vi "Magazine_Hardware_Begin.vi"(8 "error in":errorcluster) -> (0 "error out":errorcluster)   [LabVIEW 2020]
uses:
  <vilib>/Rock Robotics/SystemInterfaces/AI/FPGA_AIChannel.ctl
  <vilib>/Rock Robotics/WPI/ThirdParty/Phoenix-LabVIEW/Motor Controller/Controls/CTRE_Phoenix_MotorControl_NeutralMode.ctl
  <vilib>/Rock Robotics/WPI/ThirdParty/Phoenix-LabVIEW/Motor Controller/Controls/CTRE_Phoenix_MotorControl_StatusFrameEnhanced.ctl
  Globals/Magazine_Globals.vi
panel:
  out "appended array":u32[](array[numeric])
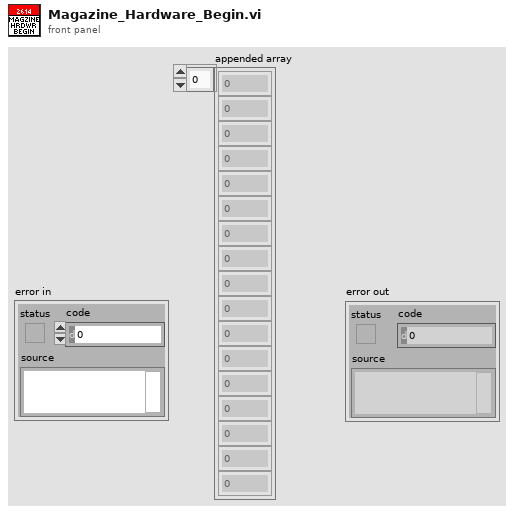
[diagram p1: front panel]
types:
  T1 = typedef "CTRE_Phoenix_MotorControl_StatusFrameEnhanced.ctl" = u16
  T2 = typedef "CTRE_Phoenix_MotorControl_NeutralMode.ctl" = enum8{"EEPROMSetting", "Override to Coast", "Override to Brake"}
  T3 = typedef "FPGA_AIChannel.ctl" = enum8{"AI 0", "AI 1", "AI 2", "AI 3", "AI MXP 0", "AI MXP 1", "AI MXP 2", "AI MXP 3", "Invalid"}
  T4 = typedef "WPI_MotorControlDeviceRef.ctl" = cluster{"DeviceStatus":errorcluster, "Type":T5, "PWM":cluster{"PWM Channel":T6, "DeadBand":T7}, "CAN":cluster{"Device Number":u8, "SetOutput VI Ref":variant, "GetOutput VI Ref":variant, "Enable VI Ref":variant, "Disable VI Ref":variant, "Data":variant}, "Invert":bool, "DIO PWM":cluster{"PWM \"Enable\" Channel":T6, "DIOChannel":T8, "PWM Rate":dbl}}
  T5 = typedef "WPI_MotorControlType.ctl" = enum16{"PWM", "CAN", "DIO PWM"}
  T6 = typedef "FPGA_DIOPWMChannel.ctl" = enum8{"PWM 0", "PWM 1", "PWM 2", "PWM 3", "PWM 4", "PWM 5", "PWM 6", "PWM 7", "PWM 8", "PWM 9", "PWM MXP 0", "PWM MXP 1", "PWM MXP 2", "PWM MXP 3", "PWM MXP 4", "PWM MXP 5", "PWM MXP 6", "PWM MXP 7", "PWM MXP 8", "PWM MXP 9", "Invalid"}
  T7 = typedef "WPI_PWMDeadband.ctl" = cluster{"Name":string, "maxPositivePwm":i32, "minPositivePwm":i32, "centerPwm":i32, "maxNegativePwm":i32, "minNegativePwm":i32, "angularRange":u16}
  T8 = typedef "FPGA_DIOChannel.ctl" = enum8{"DIO 0", "DIO 1", "DIO 2", "DIO 3", "DIO 4", "DIO 5", "DIO 6", "DIO 7", "DIO 8", "DIO 9", "DIO MXP 0", "DIO MXP 1", "DIO MXP 2", "DIO MXP 3", "DIO MXP 4", "DIO MXP 5", "DIO MXP 6", "DIO MXP 7", "DIO MXP 8", "DIO MXP 9", "DIO MXP 10", "DIO MXP 11", "DIO MXP 12", "DIO MXP 13", "DIO MXP 14", "DIO MXP 15", "SPI Port CS1", "SPI Port CS2", "SPI Port CS3", "SPI Port MISO", "SPI Port MOSI", "Invalid"}
  T9 = typedef "WPI_AnalogChannelDevRef.ctl" = cluster{"DevStatus":errorcluster, "Analog Channel":T3}
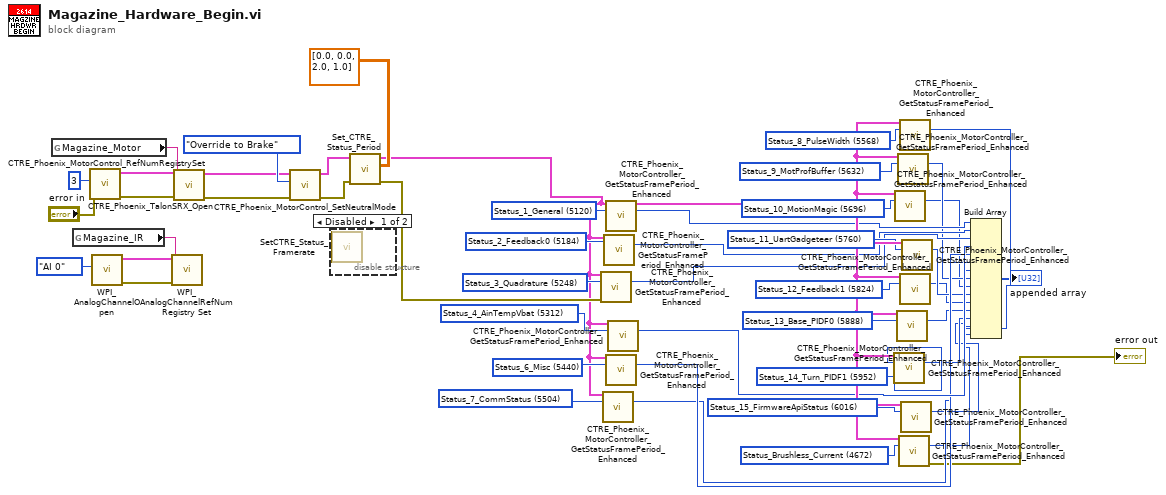
[diagram p0: block diagram]
diagram:
  w26 = T1 4672 items=["Status_1_General"=5120, "Status_2_Feedback0"=5184, "Status_3_Quadrature"=5248, "Status_4_AinTempVbat"=5312, "Status_6_Misc"=5440, "Status_7_CommStatus"=5504, "Status_8_PulseWidth"=5568, "Status_9_MotProfBuffer"=5632, "Status_10_MotionMagic"=5696, "Status_11_UartGadgeteer"=5760, "Status_12_Feedback1"=5824, "Status_13_Base_PIDF0"=5888, "Status_14_Turn_PIDF1"=5952, "Status_15_FirmwareApiStatus"=6016, "Status_Brushless_Current"=4672] ("Status Frame")
  w27 = T1 6016 items=["Status_1_General"=5120, "Status_2_Feedback0"=5184, "Status_3_Quadrature"=5248, "Status_4_AinTempVbat"=5312, "Status_6_Misc"=5440, "Status_7_CommStatus"=5504, "Status_8_PulseWidth"=5568, "Status_9_MotProfBuffer"=5632, "Status_10_MotionMagic"=5696, "Status_11_UartGadgeteer"=5760, "Status_12_Feedback1"=5824, "Status_13_Base_PIDF0"=5888, "Status_14_Turn_PIDF1"=5952, "Status_15_FirmwareApiStatus"=6016, "Status_Brushless_Current"=4672] ("Status Frame")
  w28 = T1 5952 items=["Status_1_General"=5120, "Status_2_Feedback0"=5184, "Status_3_Quadrature"=5248, "Status_4_AinTempVbat"=5312, "Status_6_Misc"=5440, "Status_7_CommStatus"=5504, "Status_8_PulseWidth"=5568, "Status_9_MotProfBuffer"=5632, "Status_10_MotionMagic"=5696, "Status_11_UartGadgeteer"=5760, "Status_12_Feedback1"=5824, "Status_13_Base_PIDF0"=5888, "Status_14_Turn_PIDF1"=5952, "Status_15_FirmwareApiStatus"=6016, "Status_Brushless_Current"=4672] ("Status Frame")
  w29 = T1 5888 items=["Status_1_General"=5120, "Status_2_Feedback0"=5184, "Status_3_Quadrature"=5248, "Status_4_AinTempVbat"=5312, "Status_6_Misc"=5440, "Status_7_CommStatus"=5504, "Status_8_PulseWidth"=5568, "Status_9_MotProfBuffer"=5632, "Status_10_MotionMagic"=5696, "Status_11_UartGadgeteer"=5760, "Status_12_Feedback1"=5824, "Status_13_Base_PIDF0"=5888, "Status_14_Turn_PIDF1"=5952, "Status_15_FirmwareApiStatus"=6016, "Status_Brushless_Current"=4672] ("Status Frame")
  w34 = T1 5824 items=["Status_1_General"=5120, "Status_2_Feedback0"=5184, "Status_3_Quadrature"=5248, "Status_4_AinTempVbat"=5312, "Status_6_Misc"=5440, "Status_7_CommStatus"=5504, "Status_8_PulseWidth"=5568, "Status_9_MotProfBuffer"=5632, "Status_10_MotionMagic"=5696, "Status_11_UartGadgeteer"=5760, "Status_12_Feedback1"=5824, "Status_13_Base_PIDF0"=5888, "Status_14_Turn_PIDF1"=5952, "Status_15_FirmwareApiStatus"=6016, "Status_Brushless_Current"=4672] ("Status Frame")
  w30 = T1 5760 items=["Status_1_General"=5120, "Status_2_Feedback0"=5184, "Status_3_Quadrature"=5248, "Status_4_AinTempVbat"=5312, "Status_6_Misc"=5440, "Status_7_CommStatus"=5504, "Status_8_PulseWidth"=5568, "Status_9_MotProfBuffer"=5632, "Status_10_MotionMagic"=5696, "Status_11_UartGadgeteer"=5760, "Status_12_Feedback1"=5824, "Status_13_Base_PIDF0"=5888, "Status_14_Turn_PIDF1"=5952, "Status_15_FirmwareApiStatus"=6016, "Status_Brushless_Current"=4672] ("Status Frame")
  w35 = T1 5696 items=["Status_1_General"=5120, "Status_2_Feedback0"=5184, "Status_3_Quadrature"=5248, "Status_4_AinTempVbat"=5312, "Status_6_Misc"=5440, "Status_7_CommStatus"=5504, "Status_8_PulseWidth"=5568, "Status_9_MotProfBuffer"=5632, "Status_10_MotionMagic"=5696, "Status_11_UartGadgeteer"=5760, "Status_12_Feedback1"=5824, "Status_13_Base_PIDF0"=5888, "Status_14_Turn_PIDF1"=5952, "Status_15_FirmwareApiStatus"=6016, "Status_Brushless_Current"=4672] ("Status Frame")
  w31 = T1 5632 items=["Status_1_General"=5120, "Status_2_Feedback0"=5184, "Status_3_Quadrature"=5248, "Status_4_AinTempVbat"=5312, "Status_6_Misc"=5440, "Status_7_CommStatus"=5504, "Status_8_PulseWidth"=5568, "Status_9_MotProfBuffer"=5632, "Status_10_MotionMagic"=5696, "Status_11_UartGadgeteer"=5760, "Status_12_Feedback1"=5824, "Status_13_Base_PIDF0"=5888, "Status_14_Turn_PIDF1"=5952, "Status_15_FirmwareApiStatus"=6016, "Status_Brushless_Current"=4672] ("Status Frame")
  w36 = T1 5568 items=["Status_1_General"=5120, "Status_2_Feedback0"=5184, "Status_3_Quadrature"=5248, "Status_4_AinTempVbat"=5312, "Status_6_Misc"=5440, "Status_7_CommStatus"=5504, "Status_8_PulseWidth"=5568, "Status_9_MotProfBuffer"=5632, "Status_10_MotionMagic"=5696, "Status_11_UartGadgeteer"=5760, "Status_12_Feedback1"=5824, "Status_13_Base_PIDF0"=5888, "Status_14_Turn_PIDF1"=5952, "Status_15_FirmwareApiStatus"=6016, "Status_Brushless_Current"=4672] ("Status Frame")
  w6 = T1 5504 items=["Status_1_General"=5120, "Status_2_Feedback0"=5184, "Status_3_Quadrature"=5248, "Status_4_AinTempVbat"=5312, "Status_6_Misc"=5440, "Status_7_CommStatus"=5504, "Status_8_PulseWidth"=5568, "Status_9_MotProfBuffer"=5632, "Status_10_MotionMagic"=5696, "Status_11_UartGadgeteer"=5760, "Status_12_Feedback1"=5824, "Status_13_Base_PIDF0"=5888, "Status_14_Turn_PIDF1"=5952, "Status_15_FirmwareApiStatus"=6016, "Status_Brushless_Current"=4672] ("Status Frame")
  w32 = T1 5440 items=["Status_1_General"=5120, "Status_2_Feedback0"=5184, "Status_3_Quadrature"=5248, "Status_4_AinTempVbat"=5312, "Status_6_Misc"=5440, "Status_7_CommStatus"=5504, "Status_8_PulseWidth"=5568, "Status_9_MotProfBuffer"=5632, "Status_10_MotionMagic"=5696, "Status_11_UartGadgeteer"=5760, "Status_12_Feedback1"=5824, "Status_13_Base_PIDF0"=5888, "Status_14_Turn_PIDF1"=5952, "Status_15_FirmwareApiStatus"=6016, "Status_Brushless_Current"=4672] ("Status Frame")
  w33 = T1 5312 items=["Status_1_General"=5120, "Status_2_Feedback0"=5184, "Status_3_Quadrature"=5248, "Status_4_AinTempVbat"=5312, "Status_6_Misc"=5440, "Status_7_CommStatus"=5504, "Status_8_PulseWidth"=5568, "Status_9_MotProfBuffer"=5632, "Status_10_MotionMagic"=5696, "Status_11_UartGadgeteer"=5760, "Status_12_Feedback1"=5824, "Status_13_Base_PIDF0"=5888, "Status_14_Turn_PIDF1"=5952, "Status_15_FirmwareApiStatus"=6016, "Status_Brushless_Current"=4672] ("Status Frame")
  w7 = T1 5248 items=["Status_1_General"=5120, "Status_2_Feedback0"=5184, "Status_3_Quadrature"=5248, "Status_4_AinTempVbat"=5312, "Status_6_Misc"=5440, "Status_7_CommStatus"=5504, "Status_8_PulseWidth"=5568, "Status_9_MotProfBuffer"=5632, "Status_10_MotionMagic"=5696, "Status_11_UartGadgeteer"=5760, "Status_12_Feedback1"=5824, "Status_13_Base_PIDF0"=5888, "Status_14_Turn_PIDF1"=5952, "Status_15_FirmwareApiStatus"=6016, "Status_Brushless_Current"=4672] ("Status Frame")
  w8 = T1 5184 items=["Status_1_General"=5120, "Status_2_Feedback0"=5184, "Status_3_Quadrature"=5248, "Status_4_AinTempVbat"=5312, "Status_6_Misc"=5440, "Status_7_CommStatus"=5504, "Status_8_PulseWidth"=5568, "Status_9_MotProfBuffer"=5632, "Status_10_MotionMagic"=5696, "Status_11_UartGadgeteer"=5760, "Status_12_Feedback1"=5824, "Status_13_Base_PIDF0"=5888, "Status_14_Turn_PIDF1"=5952, "Status_15_FirmwareApiStatus"=6016, "Status_Brushless_Current"=4672] ("Status Frame")
  w37 = T1 5120 items=["Status_1_General"=5120, "Status_2_Feedback0"=5184, "Status_3_Quadrature"=5248, "Status_4_AinTempVbat"=5312, "Status_6_Misc"=5440, "Status_7_CommStatus"=5504, "Status_8_PulseWidth"=5568, "Status_9_MotProfBuffer"=5632, "Status_10_MotionMagic"=5696, "Status_11_UartGadgeteer"=5760, "Status_12_Feedback1"=5824, "Status_13_Base_PIDF0"=5888, "Status_14_Turn_PIDF1"=5952, "Status_15_FirmwareApiStatus"=6016, "Status_Brushless_Current"=4672] ("Status Frame")
  n1 = global read "Magazine_Globals.vi" "Magazine_Motor"() -> (w50:string)
  n2 = global read "Magazine_Globals.vi" "Magazine_IR"() -> (w44:string)
  n3 = call <vilib>:"CTRE_Phoenix_TalonSRX_Open.vi"("error in"="error in", "Device Number"=u8 3) -> ("error out"=w48:errorcluster, "PhoenixMotorControlDevRef"=w49:T4)  [unwired: 8 in]
  n4 = call <vilib>:"WPI_AnalogChannelOpen.vi"("Analog Channel"=FPGA_AIChannel."AI 0") -> ("error out"=w45:errorcluster, "AIDeviceRef"=w46:T9)  [unwired: 9 in]
  n5 = call <vilib>:"WPI_AnalogChannelRefNum Registry Set.vi"("error in (no error)"=w45, "refnum name"=w44, "AIDeviceRef"=w46) -> ()  [unwired: 7 in, 2 out]
  n6 = call <vilib>:"CTRE_Phoenix_MotorControl_RefNumRegistrySet.vi"("error in (no error)"=w48, "refnum name"=w50, "PhoenixMotorControlDevRef"=w49) -> ("error out"=w39:errorcluster, "PhoenixMotorControlDevRef"=w40:T4)  [unwired: 7 in]
  n7 = call <vilib>:"CTRE_Phoenix_MotorControl_SetNeutralMode.vi"("error in (no error)"=w39, "Motor Control Neutral Mode"=CTRE_Phoenix_MotorControl_NeutralMode."Override to Brake", "PhoenixMotorControlDevRef"=w40) -> ("error out"=w3:errorcluster, "PhoenixMotorControlDevRef"=w4:T4)  [unwired: 7 in]
  n8 = disable-structure shown="Disabled" {
    frame Disabled {
      n9 = call "SetCTRE_Status_Framerate.vi"() -> ()  [unwired: 10 in, 2 out]
    }
    frame Enabled {
    }
  }
  n10 = call "Set_CTRE_Status_Period.vi"("error in (no error)"=w3, "Frame Settings"=dbl[][] [[0.0], [0.0], [2.0], [1.0]], "PhoenixMotorControlDevRef"=w4) -> ("error out"=w2:errorcluster, "PhoenixMotorControlDevRef 2"=w1:T4)  [unwired: 7 in]
  n11 = call <vilib>:"CTRE_Phoenix_MotorController_GetStatusFramePeriod_Enhanced.vi"("PhoenixMotorControlDevRef"=w1, "Status Frame"=w7, "error in"=w2) -> ("periodMs"=w23:u32)  [unwired: 10 in, 2 out]
  n12 = call <vilib>:"CTRE_Phoenix_MotorController_GetStatusFramePeriod_Enhanced.vi"("PhoenixMotorControlDevRef"=w1, "Status Frame"=w6) -> ("periodMs"=w20:u32)  [unwired: 11 in, 2 out]
  n13 = call <vilib>:"CTRE_Phoenix_MotorController_GetStatusFramePeriod_Enhanced.vi"("PhoenixMotorControlDevRef"=w1, "Status Frame"=w8) -> ("periodMs"=w24:u32)  [unwired: 11 in, 2 out]
  n14 = call <vilib>:"CTRE_Phoenix_MotorController_GetStatusFramePeriod_Enhanced.vi"("PhoenixMotorControlDevRef"=w1, "Status Frame"=w37) -> ("PhoenixMotorControlDevRef"=w38:T4, "periodMs"=w25:u32)  [unwired: 11 in, 1 out]
  n15 = call <vilib>:"CTRE_Phoenix_MotorController_GetStatusFramePeriod_Enhanced.vi"("PhoenixMotorControlDevRef"=w1, "Status Frame"=w32) -> ("periodMs"=w21:u32)  [unwired: 11 in, 2 out]
  n16 = call <vilib>:"CTRE_Phoenix_MotorController_GetStatusFramePeriod_Enhanced.vi"("PhoenixMotorControlDevRef"=w1, "Status Frame"=w33) -> ("periodMs"=w22:u32)  [unwired: 11 in, 2 out]
  n17 = call <vilib>:"CTRE_Phoenix_MotorController_GetStatusFramePeriod_Enhanced.vi"("PhoenixMotorControlDevRef"=w38, "Status Frame"=w28) -> ("periodMs"=w13:u32)  [unwired: 11 in, 2 out]
  n18 = call <vilib>:"CTRE_Phoenix_MotorController_GetStatusFramePeriod_Enhanced.vi"("PhoenixMotorControlDevRef"=w38, "Status Frame"=w35) -> ("periodMs"=w17:u32)  [unwired: 11 in, 2 out]
  n19 = call <vilib>:"CTRE_Phoenix_MotorController_GetStatusFramePeriod_Enhanced.vi"("PhoenixMotorControlDevRef"=w38, "Status Frame"=w29) -> ("periodMs"=w14:u32)  [unwired: 11 in, 2 out]
  n20 = call <vilib>:"CTRE_Phoenix_MotorController_GetStatusFramePeriod_Enhanced.vi"("PhoenixMotorControlDevRef"=w38, "Status Frame"=w31) -> ("periodMs"=w18:u32)  [unwired: 11 in, 2 out]
  n21 = call <vilib>:"CTRE_Phoenix_MotorController_GetStatusFramePeriod_Enhanced.vi"("PhoenixMotorControlDevRef"=w38, "Status Frame"=w26) -> ("periodMs"=w11:u32, "error out"=→"error out":errorcluster)  [unwired: 11 in, 1 out]
  n22 = call <vilib>:"CTRE_Phoenix_MotorController_GetStatusFramePeriod_Enhanced.vi"("PhoenixMotorControlDevRef"=w38, "Status Frame"=w36) -> ("periodMs"=w19:u32)  [unwired: 11 in, 2 out]
  n23 = call <vilib>:"CTRE_Phoenix_MotorController_GetStatusFramePeriod_Enhanced.vi"("PhoenixMotorControlDevRef"=w38, "Status Frame"=w34) -> ("periodMs"=w15:u32)  [unwired: 11 in, 2 out]
  n24 = call <vilib>:"CTRE_Phoenix_MotorController_GetStatusFramePeriod_Enhanced.vi"("PhoenixMotorControlDevRef"=w38, "Status Frame"=w27) -> ("periodMs"=w12:u32)  [unwired: 11 in, 2 out]
  n25 = call <vilib>:"CTRE_Phoenix_MotorController_GetStatusFramePeriod_Enhanced.vi"("PhoenixMotorControlDevRef"=w38, "Status Frame"=w30) -> ("periodMs"=w16:u32)  [unwired: 11 in, 2 out]
  n26 = Build Array(w25, w24, w23, w22, w21, w20, w19, w18, w17, w16, w15, w14, w13, w12, w11) -> (→"appended array":u32[])
